vi "Temp Encoder Data.vi"() -> ()   [LabVIEW 2013]
panel:
  in  "Left Encoder Temp Data":cluster{dbl, "String":string}
  in  "Right Encoder Temp Data":cluster{dbl, "String":string}
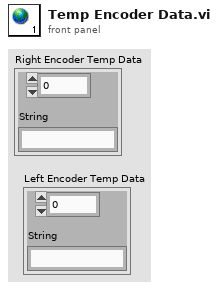
[diagram p1: front panel]
diagram:
